vi "quotient.vi"(2 "Y":dbl, 3 "Nearest?":bool=TRUE, 4 "X":dbl) -> (0 "s? t:f":dbl, 1 "x = y?":bool)   [LabVIEW 2015]
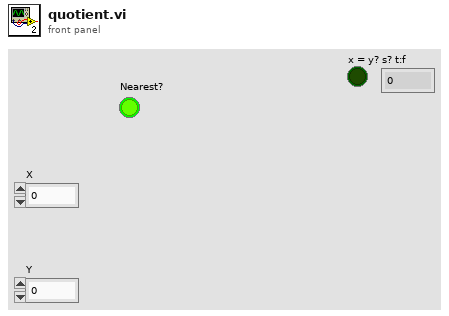
[diagram p1: front panel]
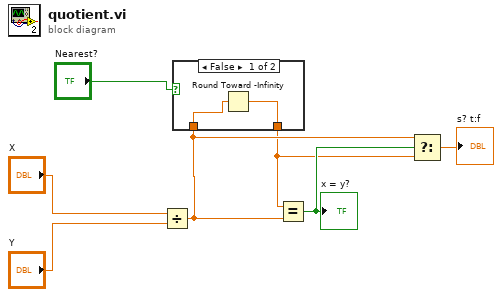
[diagram p0: block diagram]
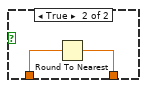
[diagram p2: hidden frame]
diagram:
  n1 = Divide(x="X", y="Y") -> (x/y=w4:dbl)
  n2 = case shown="False" "Nearest?" {
    tunnel: w4 -> [w9 w11]
    tunnel: [w8 w10] -> w3
    frame False {
      n3 = Round Toward -Infinity(1:w9) -> (0:w8:dbl)
    }
    frame True {
      n4 = Round To Nearest(number=w11) -> (nearest integer value=w10:dbl)
    }
  }
  n5 = Equal?(x=w3, y=w4) -> (x = y?=w5:bool)
  "x = y?" <- w5
  n6 = Select(t=w4, s=w5, f=w3) -> (s? t:f=→"s? t:f":dbl)
